vi "Tornado.vi"(11 "VI Ref":refnum<vi>) -> ()   [LabVIEW 2019]
doc: "Tornado disaster. A tornado appears on the left edge of the screen and then travels right across the screen. It will place any objects it passes close by into a spin, messing up block diagram wiring. There's also a 15% chance it will destroy an object on contact."
uses:
  _Sound/Music Player Command Message.ctl
  _Sound/Music Player Command.ctl
  _2D/Point.ctl
  <vilib>/Utility/miscctls.llb/LVRectTypeDef.ctl
  <vilib>/Utility/miscctls.llb/LVPositionTypeDef.ctl
  _SubVIs/Tornado State Enum.ctl
  <vilib>/numeric/Random Number (Range) U64.vi
  <vilib>/numeric/Random Number (Range) I64.vi
  <vilib>/numeric/Random Number (Range) DBL.vi
  <vilib>/numeric/sub_Random U32.vi
  _Window/Window.lvlib
  _Sound/Sound.lvlib
  _2D/2D.lvlib
panel:
  out "Tornado":u16(ring)
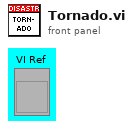
[diagram p1: front panel]
types:
  T1 = typedef "Tornado State Enum.ctl" = enum16{"Init", "Init Window", "Play Music", "Fade In Window", "Update Time", "Update Window Position", "Check Window Over BD", "Object Collision Detection", "Move Objects", "Update Graphic", "Fade Out Window", "Close Window"}
  T2 = typedef "LVPositionTypeDef.ctl" = cluster{"Left":i32, "Top":i32}
  T3 = cluster{"Object Ref":refnum<vi>, "hWnd":i32, "Initial Time (s)":dbl, "Release Time (s)":dbl, "Center Position":T2, "Start Position":T2, "Spin Velocity":dbl}[]
  T4 = enum32{"Invalid", "Standard", "Closed", "Hidden", "Minimized", "Maximized"}
  T5 = typedef "LVRectTypeDef.ctl" = cluster{"Left":i16, "Top":i16, "Right":i16, "Bottom":i16}
  T6 = typedef "2D.lvlib/Point.ctl" = cluster{"X":i16, "Y":i16}
  T7 = typedef "Sound.lvlib/Music Player Command Message.ctl" = cluster{"Command":T8, "Data":variant}
  T8 = typedef "Sound.lvlib/Music Player Command.ctl" = enum16{"Enable", "Play", "Play Random", "Stop", "Shutdown"}
  T9 = cluster{"Object Ref":refnum<vi>, "hWnd":i32, "Initial Time (s)":dbl, "Release Time (s)":dbl, "Center Position":T2, "Start Position":T2, "Spin Velocity":dbl}
  T10 = cluster{"BDWin.NativeWindow":u64, "vi reference":refnum<vi>}[]
  T11 = typedef "LVPointTypeDef.ctl" = cluster{"Horizontal":i16, "Vertical":i16}
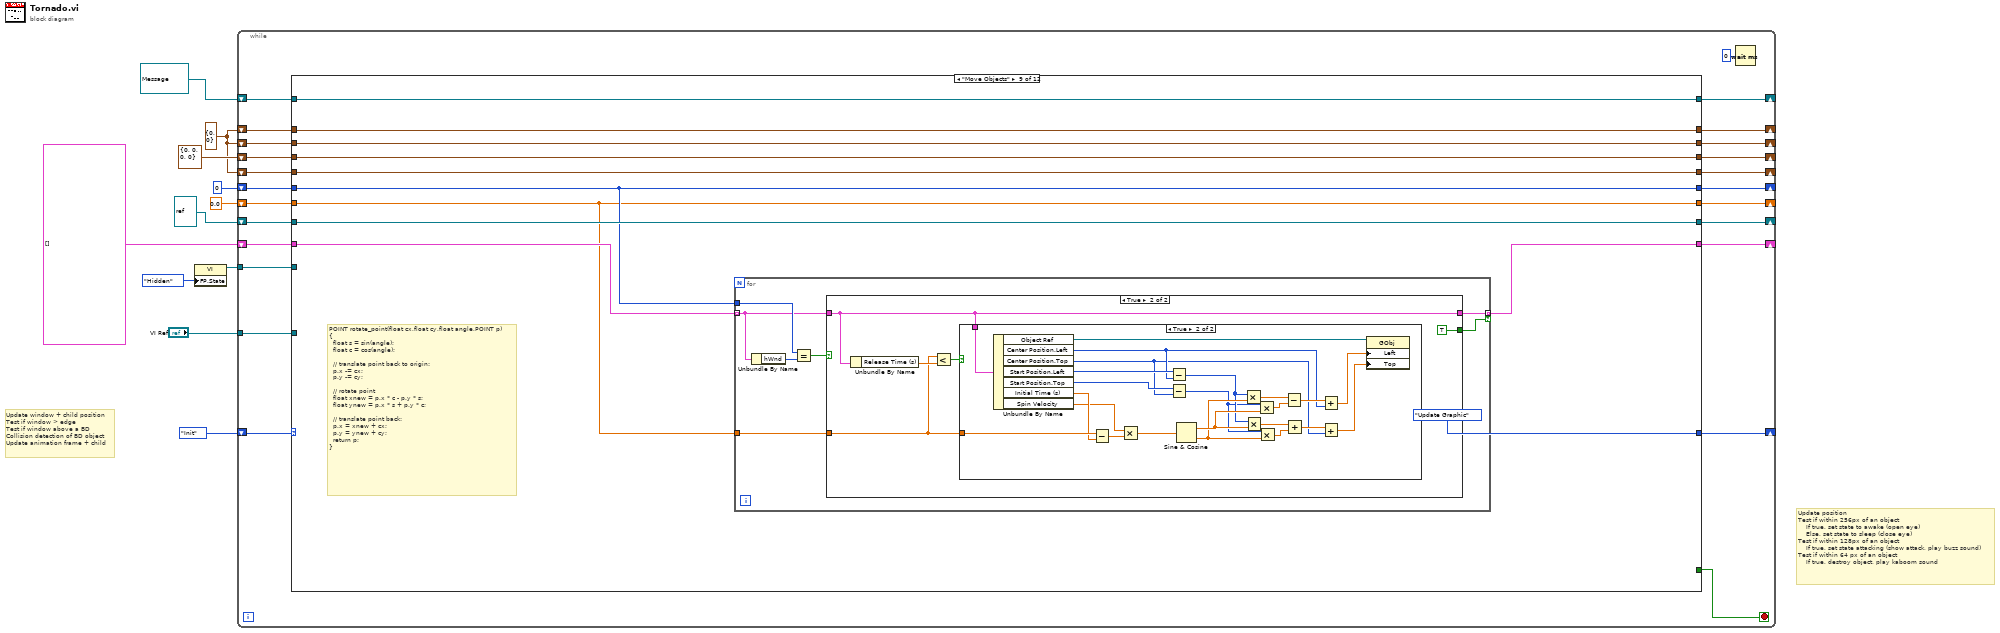
[diagram p0: block diagram]
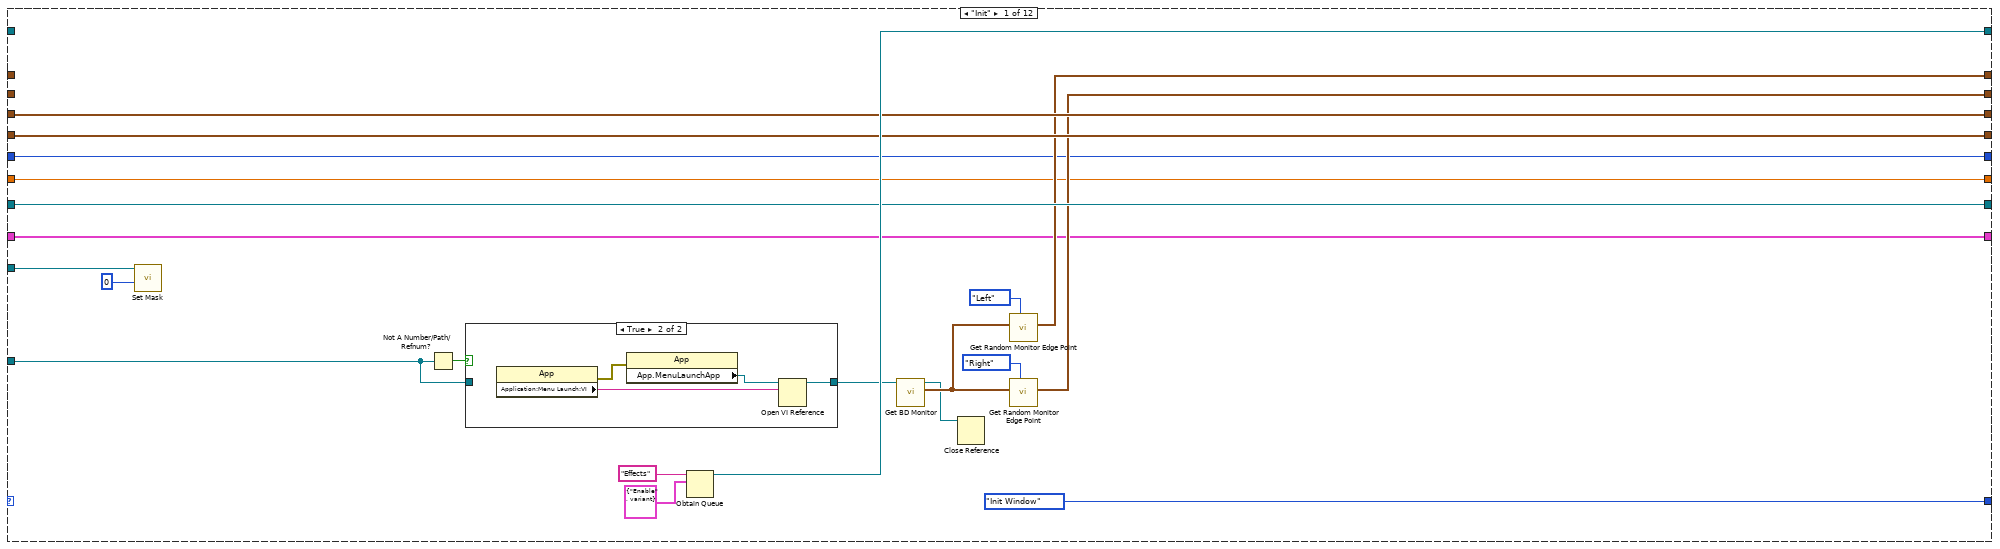
[diagram p2: hidden frame]
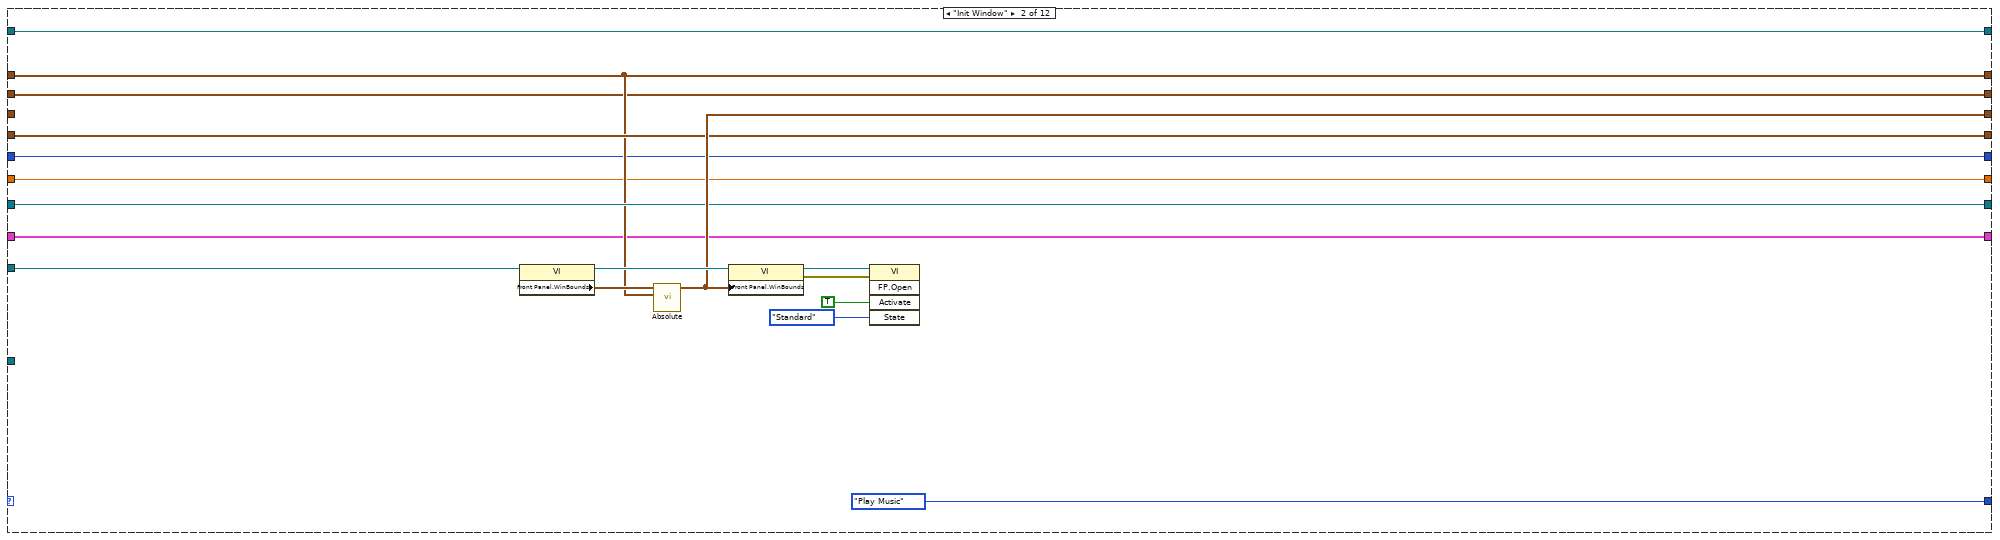
[diagram p4: hidden frame]
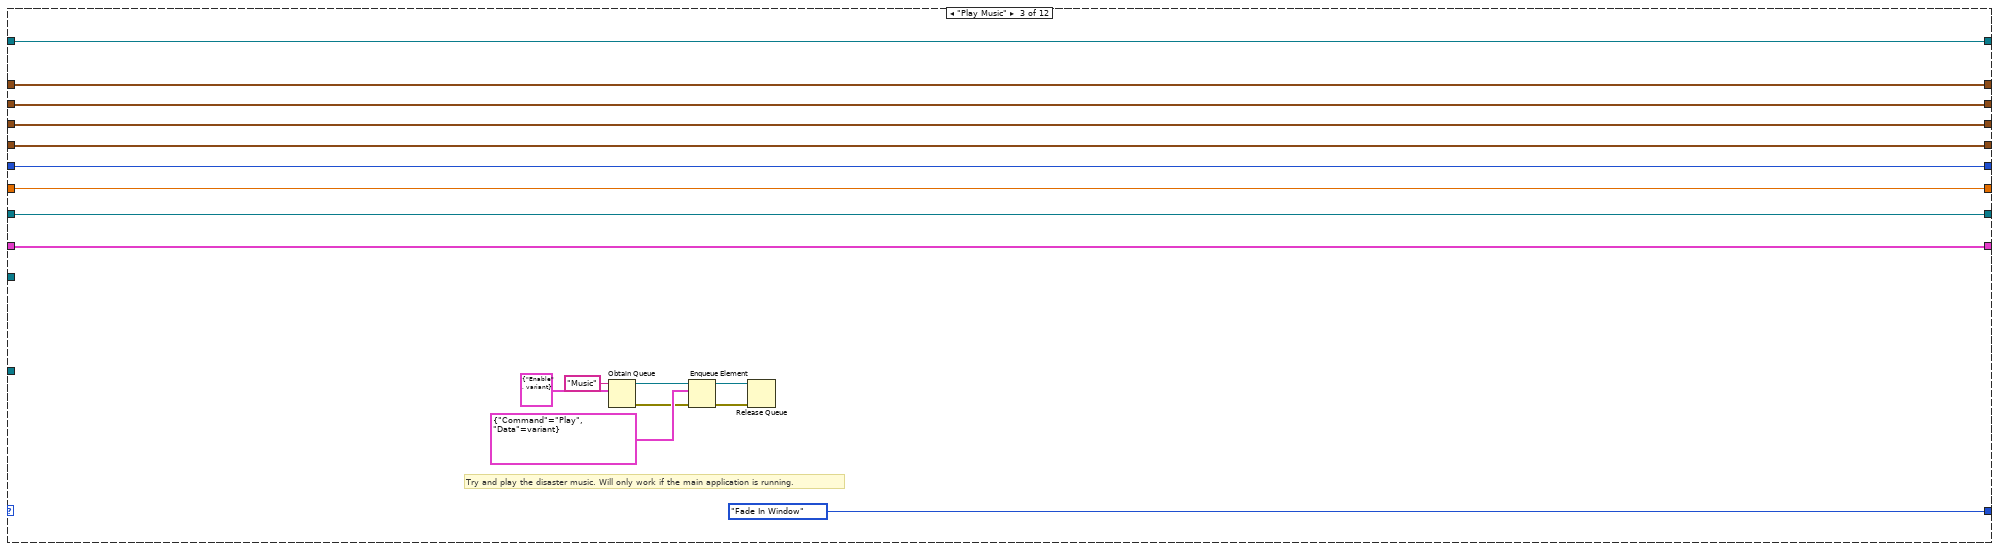
[diagram p5: hidden frame]
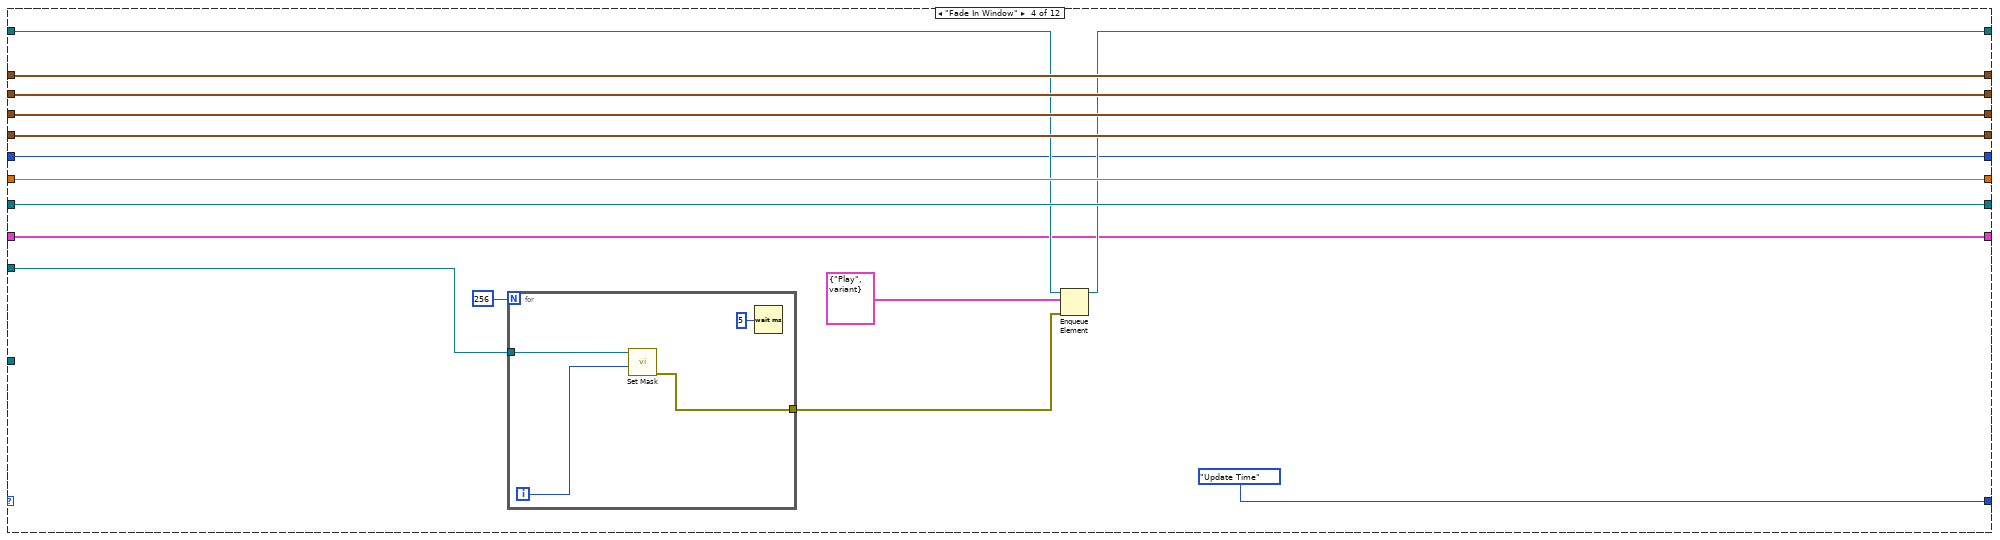
[diagram p6: hidden frame]
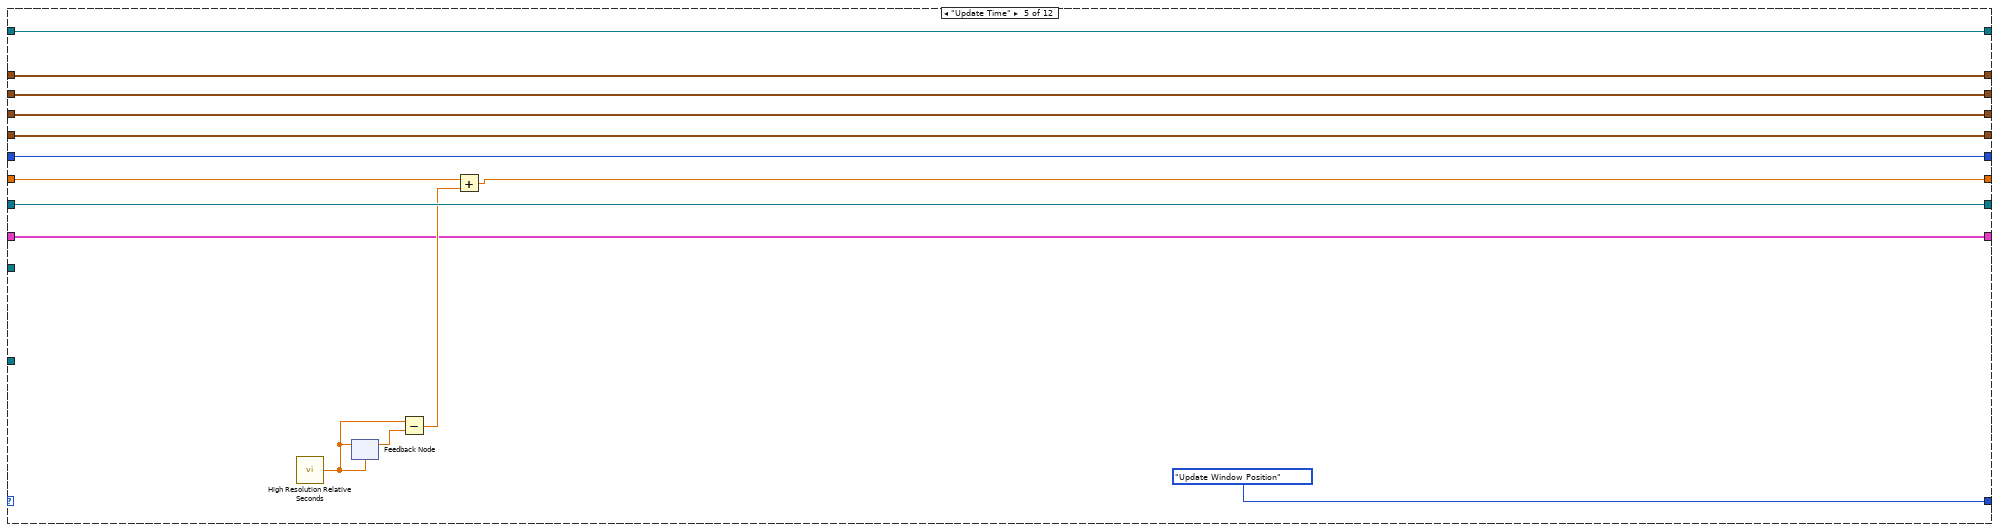
[diagram p7: hidden frame]
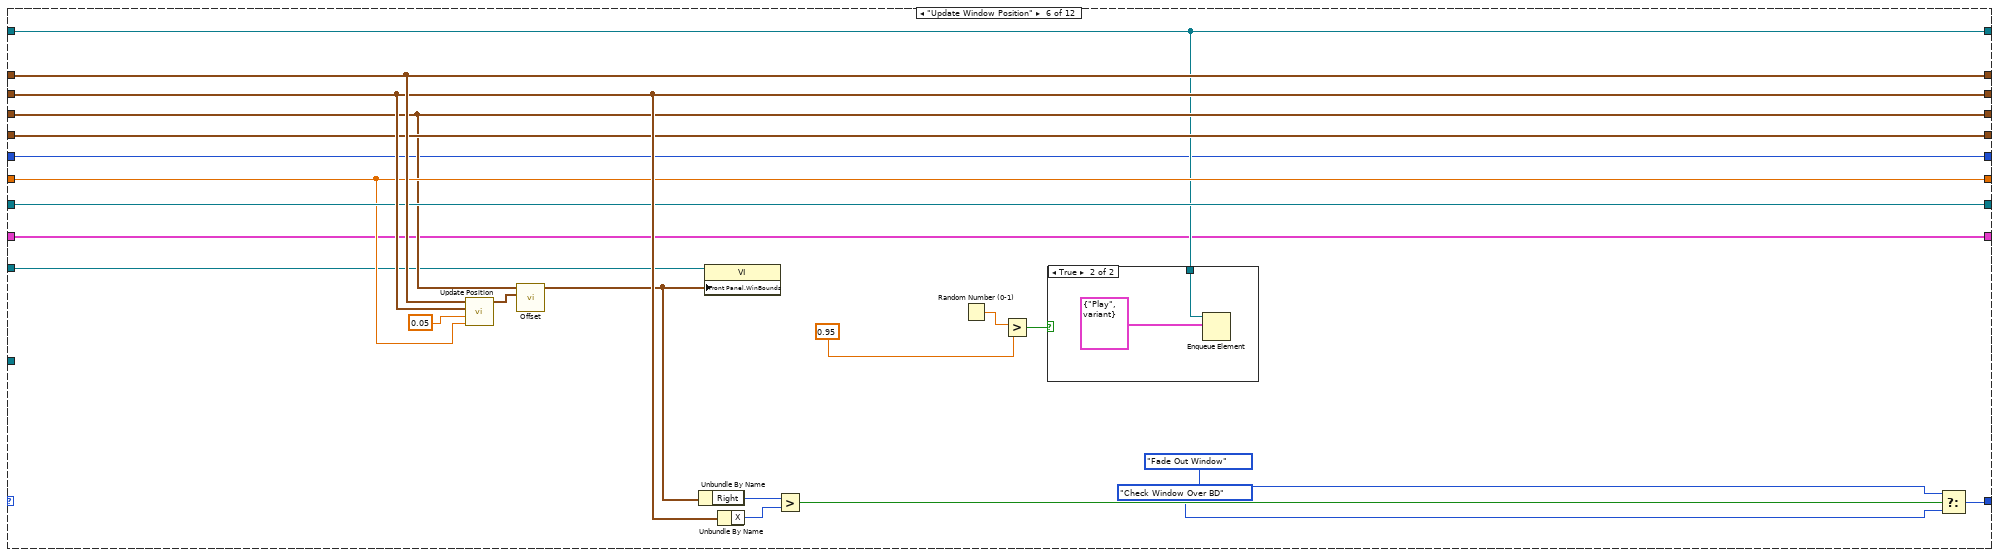
[diagram p8: hidden frame]
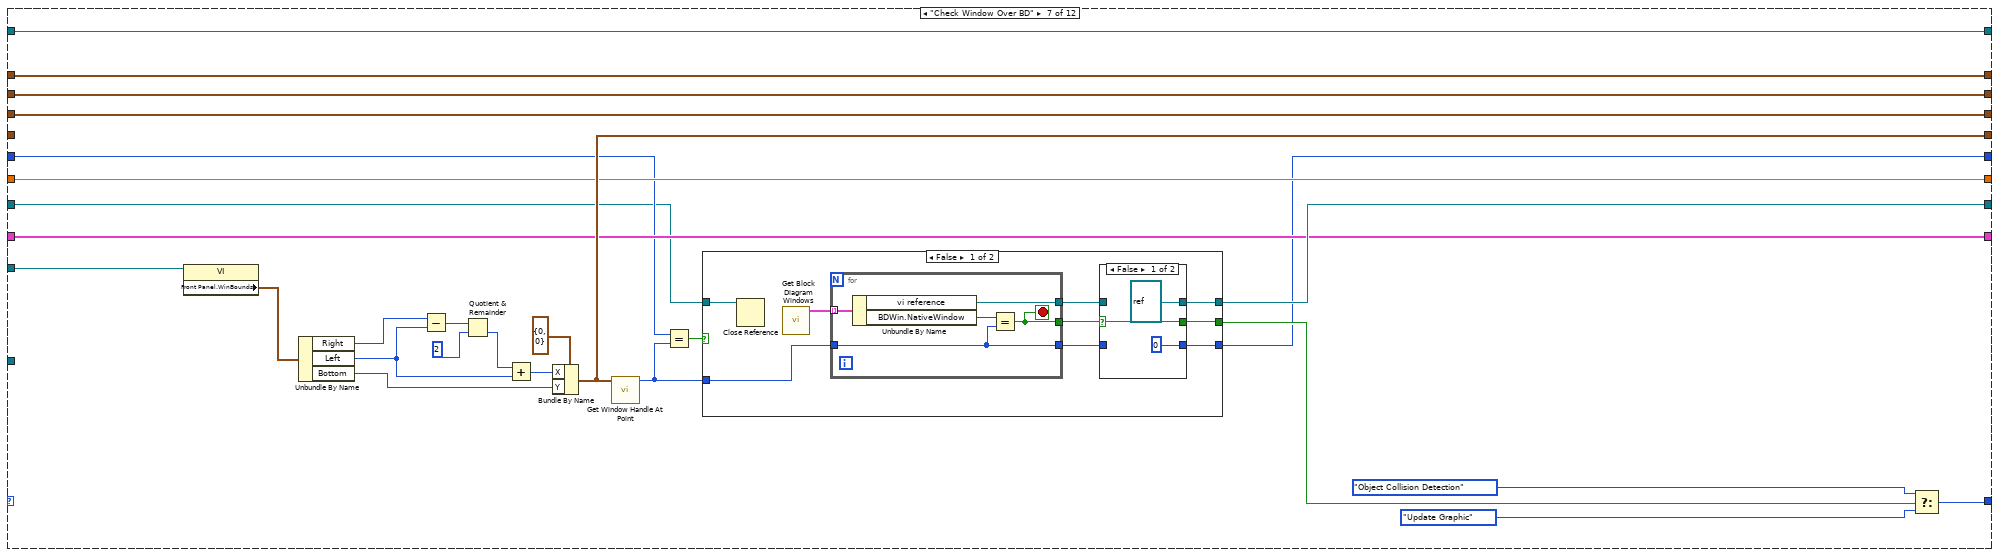
[diagram p10: hidden frame]
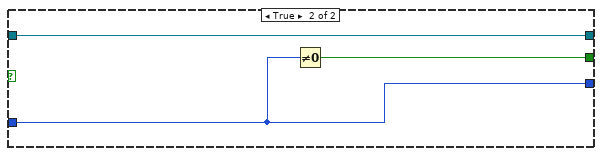
[diagram p12: hidden frame]
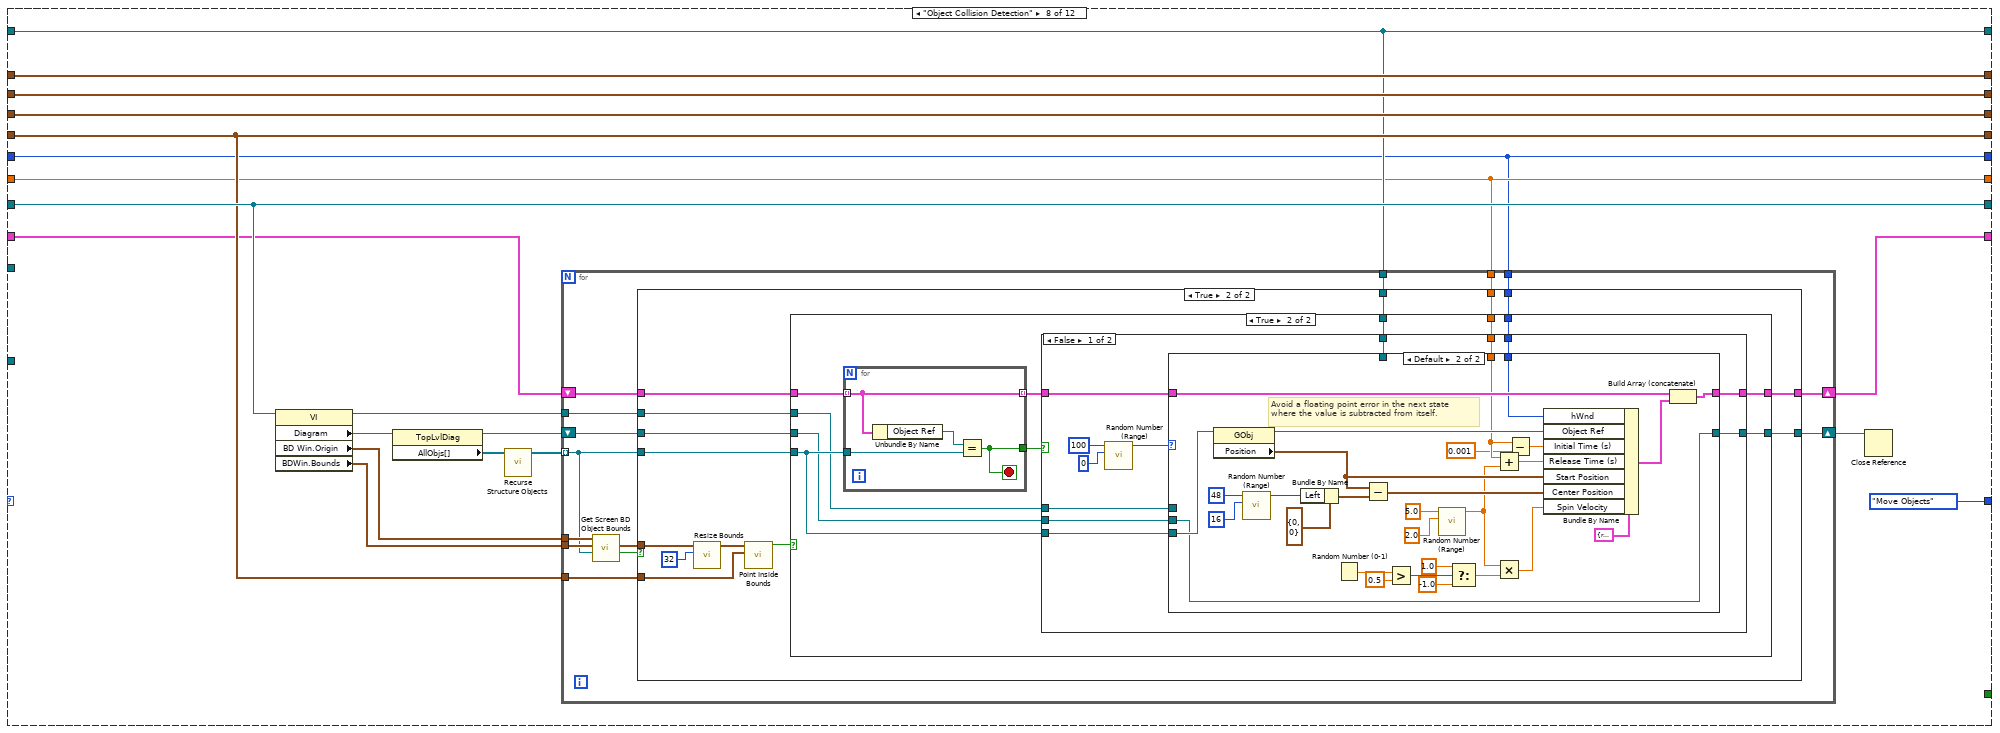
[diagram p13: hidden frame]
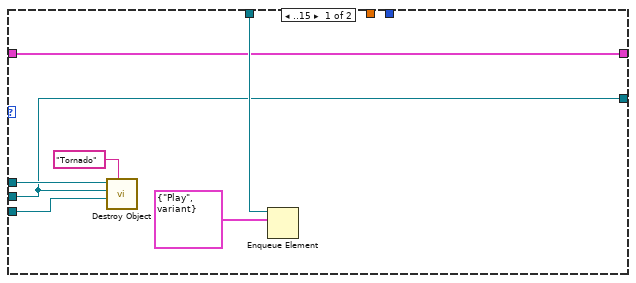
[diagram p16: hidden frame]
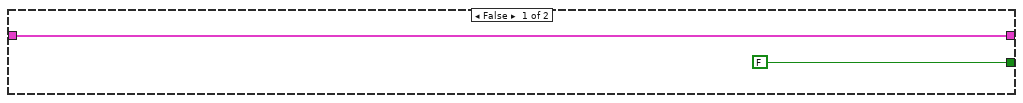
[diagram p18: hidden frame]
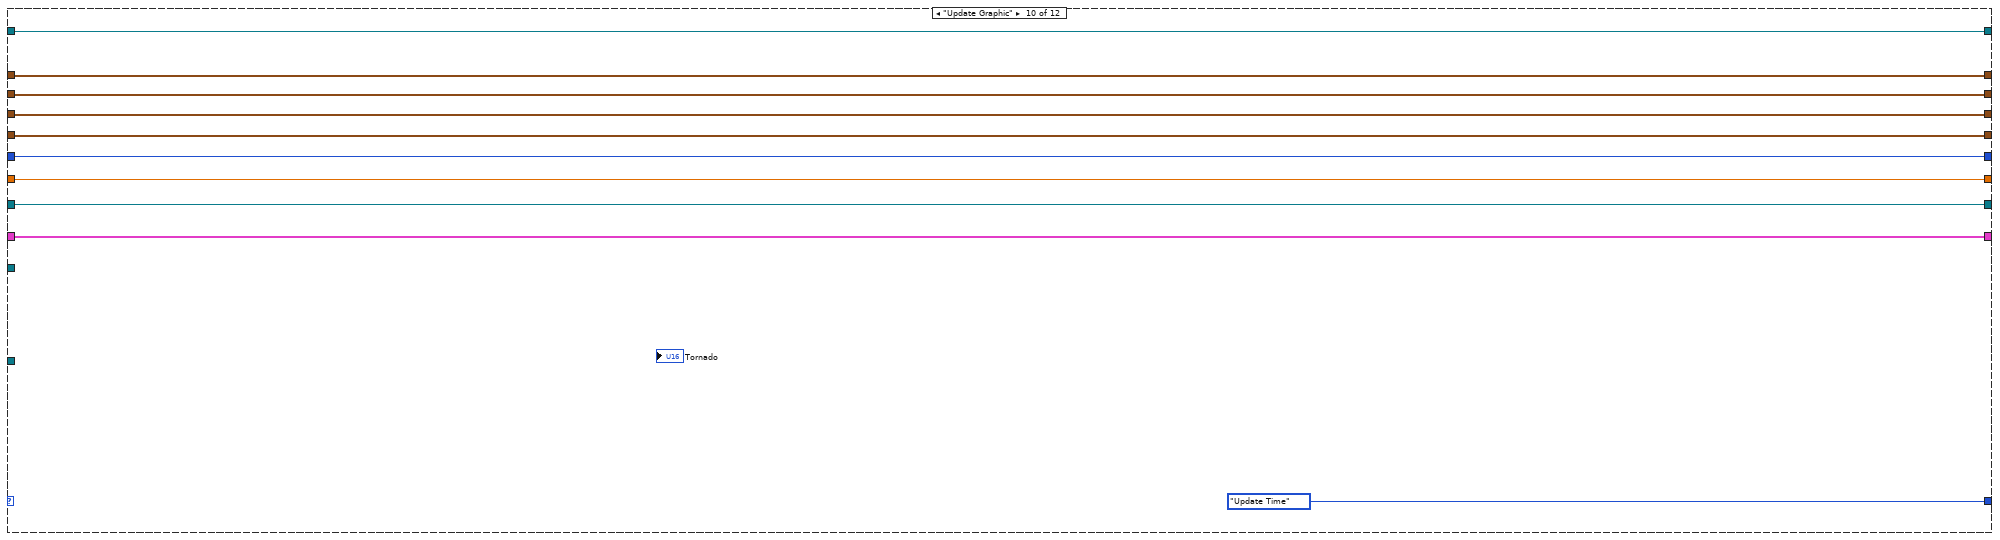
[diagram p20: hidden frame]
diagram:
  w8 = T6 {"X"=0, "Y"=0} ("Point")
  # "Update position\nTest if within 256px of an object\n    If true, set state to awake (open eye)\n    Else, set state to sleep (close eye)\nTest if within 128px of an object\n    If true, set state attacking (show attack, play buzz sound)\nTest if within 64 px of an object\n    If true, destroy object, play kaboom sound"
  # "Update window + child position\nTest if window > edge\nTest if window above a BD\nCollision detection of BD object\nUpdate animation frame + child"
  n1 = property class="VI"("FP.State"=T4."Hidden" ("Front Panel Window:State")) -> (reference out=w5:refnum<vi>)  [unwired: 2 in, 1 out]
  n2 = while {
    shift-right: [w32] -> _
    shift-left: Tornado_State_Enum."Init" ("Enum") -> [w35]
    tunnel: w5 -> [w31]
    shift-right: [w33] -> _
    shift-left: refnum<queue> refnum ("queue out") -> [w30]
    shift-right: [w29] -> _
    shift-left: w8 -> [w27]
    shift-right: [w28] -> _
    shift-left: w8 -> [w26]
    shift-right: [w25] -> _
    shift-left: T5 {"Left"=0, "Top"=0, "Right"=0, "Bottom"=0} ("Bounds Out") -> [w24]
    shift-right: [w23] -> _
    shift-left: refnum<vi> refnum ("vi reference") -> [w20]
    shift-right: [w22] -> _
    shift-left: w8 -> [w21]
    tunnel: "VI Ref" -> [w34]
    shift-right: [w17] -> _
    shift-left: 0.0 -> [w18]
    shift-right: [w14] -> _
    shift-left: T3 [] -> [w15]
    shift-right: [w13] -> _
    shift-left: 0 ("hWnd") -> [w12]
    stop <- w19 stop-if-true
    n3 = case shown="\"Move Objects\"" w35 {
      tunnel: w34 -> [w54 _ _ _ _ _ _ _ _ _ _ _]
      tunnel: [w52 w72 w89 w101 w128 w133 w179 w209 w329 w376 w388 refnum<queue> refnum ("queue out")] -> w33
      tunnel: [Tornado_State_Enum."Init Window" ("Enum") Tornado_State_Enum."Play Music" ("Enum") Tornado_State_Enum."Fade In Window" ("Enum") Tornado_State_Enum."Update Time" ("Enum") Tornado_State_Enum."Update Window Position" ("Enum") w144 w164 Tornado_State_Enum."Move Objects" ("Enum") Tornado_State_Enum."Update Graphic" ("Enum") Tornado_State_Enum."Update Time" ("Enum") Tornado_State_Enum."Close Window" ("Enum") Tornado_State_Enum."Close Window" ("Enum")] -> w32
      tunnel: w31 -> [w40 w73 _ w104 _ w138 w167 _ _ _ w381 w404]
      tunnel: w30 -> [_ w72 w89 w100 w128 w133 w179 w209 w329 w376 w388 w403]
      tunnel: [w44 w68 w88 w109 w127 w146 w178 w221 w328 w375 w387 w408] -> w29
      tunnel: [w43 w67 w87 w108 w126 w143 w177 w220 w327 w374 w386 w407] -> w28
      tunnel: w27 -> [_ w68 w88 w109 w127 w146 w178 w221 w328 w375 w387 w408]
      tunnel: w26 -> [_ w67 w87 w108 w126 w143 w177 w220 w327 w374 w386 w407]
      tunnel: [w51 w71 w86 w107 w125 w139 w176 w219 w326 w373 w385 w406] -> w25
      tunnel: w24 -> [w51 _ w86 w107 w125 w139 w176 w219 w326 w373 w385 w406]
      tunnel: [w49 w69 w84 w105 w124 w141 w163 w213 w325 w372 w384 refnum<vi> refnum ("vi reference")] -> w23
      tunnel: [w50 w70 w85 w106 w123 w142 w162 w212 w320 w371 w383 w405] -> w22
      tunnel: w21 -> [w50 w70 w85 w106 w123 w142 _ w212 w320 w371 w383 w405]
      tunnel: w20 -> [w49 w69 w84 w105 w124 w141 w153 w213 w325 w372 w384 w396]
      tunnel: [_ _ _ _ _ _ _ _ _ _ _ TRUE] -> w19
      tunnel: w18 -> [w42 w66 w83 w103 w121 w140 w161 w208 w319 w370 w380 w400]
      tunnel: [w42 w66 w83 w103 w118 w140 w161 w208 w319 w370 w380 w400] -> w17
      tunnel: w15 -> [w39 w64 w82 w98 w117 w132 w160 w206 w322 w369 w379 w399]
      tunnel: [w39 w64 w82 w98 w117 w132 w160 w207 w321 w369 w379 w399] -> w14
      tunnel: [w37 w62 w80 w96 w115 w129 w157 w204 w323 w367 w377 w397] -> w13
      tunnel: w12 -> [w37 w62 w80 w96 w115 w129 w156 w204 w323 w367 w377 w397]
      frame "Init" {
        n4 = call "Set Mask.vi"("Alpha (255)"=0, "VI Ref In"=w40) -> ()  [unwired: 8 in, 2 out]
        n5 = Not A Number/Path/Refnum?(number/path/refnum=w54) -> (NaN/Path/Refnum?=w53:bool)
        n6 = case shown="True" w53 {
          tunnel: w54 -> [w57 _]
          tunnel: [w57 w60] -> w45
          frame False {
          }
          frame True {
            n7 = property class="App"() -> (error out=w59:errorcluster, "Application:Menu Launch:VI"=w61:string)  [unwired: 2 in, 1 out]
            n8 = property class="App"(error in=w59) -> ("App.MenuLaunchApp"=w58:refnum<vi>)  [unwired: 1 in, 2 out]
            n9 = Open VI Reference(application reference (local)=w58, vi path=w61) -> (vi reference=w60:refnum<vi>)  [unwired: 4 in, 1 out]
          }
        }
        n10 = Obtain Queue(name (unnamed)="Effects", element data type=T7 {"Command"=enum."Enable", "Data"=variant} ("Message")) -> (queue out=w52:refnum<queue>)  [unwired: 3 in, 2 out]
        n11 = call "Get BD Monitor.vi"("VI Ref In"=w45) -> ("Monitor Bounds"=w48:T5, "VI Ref Out"=w36:refnum<vi>)  [unwired: 8 in, 1 out]
        n12 = Close Reference(reference=w36) -> ()  [unwired: 1 in, 1 out]
        n13 = call "Get Random Monitor Edge Point.vi"("Edge"=enum16{"Left", "Top", "Right", "Bottom"}."Left", "Monitor Bounds"=w48) -> ("Point"=w44:T6)  [unwired: 9 in]
        n14 = call "Get Random Monitor Edge Point.vi"("Edge"=enum16{"Left", "Top", "Right", "Bottom"}."Right", "Monitor Bounds"=w48) -> ("Point"=w43:T6)  [unwired: 9 in]
      }
      frame "Init Window" {
        n15 = property class="VI"(reference=w73) -> (reference out=w76:refnum<vi>, "Front Panel.WinBounds"=w78:T5)  [unwired: 1 in, 1 out]
        n16 = call "Absolute.vi"("Point"=w68, "Bounds In"=w78) -> ("Bounds Out"=w71:T5)  [unwired: 9 in]
        n17 = property class="VI"(reference=w76, "Front Panel.WinBounds"=w71) -> (reference out=w77:refnum<vi>, error out=w65:errorcluster)  [unwired: 1 in]
        n18 = invoke class="VI" method="FP.Open"(reference=w77, error in=w65, "Activate"=TRUE ("Activate?"), "State"=T4."Standard") -> ()  [unwired: 1 in, 5 out]
      }
      frame "Play Music" {
        # "Try and play the disaster music. Will only work if the main application is running."
        n19 = Obtain Queue(name (unnamed)="Music", element data type=T7 {"Command"=enum."Enable", "Data"=variant} ("Message")) -> (queue out=w92:refnum<queue>, error out=w79:errorcluster)  [unwired: 3 in, 1 out]
        n20 = Enqueue Element(queue=w92, element=T7 {"Command"=enum."Play", "Data"=variant(string "Disasters\\Disaster Decision")}, error in (no error)=w79) -> (queue out=w91:refnum<queue>, error out=w90:errorcluster)  [unwired: 1 in, 1 out]
        n21 = Release Queue(queue=w91, error in (no error)=w90) -> ()  [unwired: 1 in, 3 out]
      }
      frame "Fade In Window" {
        n22 = for {
          N: 256 -> [_]
          tunnel: w104 -> [w112]
          tunnel: [w111] -> w99
          i -> [w113]
          n23 = call "Set Mask.vi"("Alpha (255)"=w113, "VI Ref In"=w112) -> ("error out"=w111:errorcluster)  [unwired: 8 in, 1 out]
          n24 = Wait (ms)(milliseconds to wait=u32 5) -> ()  [unwired: 1 out]
        }
        n25 = Enqueue Element(queue=w100, element=T7 {"Command"=enum."Play", "Data"=variant(string "siren")}, error in (no error)=w99) -> (queue out=w101:refnum<queue>)  [unwired: 1 in, 2 out]
      }
      frame "Update Time" {
        n26 = call <vilib>:"High Resolution Relative Seconds.vi"() -> ("relative seconds"=w119:dbl)
        n27 = feedback-in #1(w119) -> ()
        n28 = feedback #1(w119) -> (w122:dbl)
        n29 = Subtract(x=w119, y=w122) -> (x-y=w120:dbl)
        n30 = Add(x=w121, y=w120) -> (x+y=w118:dbl)
      }
      frame "Update Window Position" {
        n31 = call "Update Position.vi"("Time"=w140, "Speed"=0.05 ("Speed (px/sec)"), "End Pos"=w143, "Start Pos"=w146) -> ("Current Pos"=w148:T6)  [unwired: 7 in]
        n32 = call "Offset.vi"("Point"=w148, "Bounds In"=w139) -> ("Bounds Out"=w137:T5)  [unwired: 9 in]
        n33 = Unbundle By Name(w137) -> ("Right"=w150:i16)
        n34 = property class="VI"(reference=w138, "Front Panel.WinBounds"=w137) -> ()  [unwired: 1 in, 2 out]
        n35 = Unbundle By Name(w143) -> ("X"=w149:i16)
        n36 = Greater?(x=w150, y=w149) -> (0:w145:bool)
        n37 = Random Number (0-1)() -> (number: 0 to 1=w136:dbl)
        n38 = Greater?(x=w136, y=0.95) -> (0:w134:bool)
        n39 = case shown="True" w134 {
          tunnel: w133 -> [_ w151]
          frame False {
          }
          frame True {
            n40 = Enqueue Element(queue=w151, element=T7 {"Command"=enum."Play", "Data"=variant(string "wind")}) -> ()  [unwired: 2 in, 3 out]
          }
        }
        n41 = Select(t=Tornado_State_Enum."Fade Out Window" ("Enum"), s=w145, f=Tornado_State_Enum."Check Window Over BD" ("Enum")) -> (s? t:f=w144:T1)
      }
      frame "Check Window Over BD" {
        n42 = property class="VI"(reference=w167) -> ("Front Panel.WinBounds"=w166:T5)  [unwired: 1 in, 2 out]
        n43 = Unbundle By Name(w166) -> ("Right"=w175:i16, "Left"=w171:i16, "Bottom"=w168:i16)
        n44 = Subtract(x=w175, y=w171) -> (x-y=w174:i16)
        n45 = Quotient & Remainder(x=w174, y=i16 2) -> (floor(x/y)=w172:i16)  [unwired: 1 out]
        n46 = Add(x=w172, y=w171) -> (x+y=w169:i16)
        n47 = Bundle By Name(cluster=T6 {"X"=0, "Y"=0} ("Point"), "X"=w169, "Y"=w168) -> (w162:T6)
        n48 = call "Get Window Handle At Point.vi"("Point"=w162) -> ("hWnd"=w155:i32)  [unwired: 9 in, 1 out]
        n49 = Equal?(x=w156, y=w155) -> (x = y?=w154:bool)
        n50 = case shown="False" w154 {
          tunnel: w155 -> [w187 w200]
          tunnel: [w184 w201] -> w165
          tunnel: [w181 w202] -> w163
          tunnel: [w180 w200] -> w157
          tunnel: w153 -> [w186 w202]
          frame False {
            n51 = Close Reference(reference=w186) -> ()  [unwired: 1 in, 1 out]
            n52 = call "Get Block Diagram Windows.vi"() -> ("VIs With Open BDs"=w188:T10)  [unwired: 11 in]
            n53 = for {
              tunnel: w188 -> [w199] mode=indexing
              tunnel: [w198] -> w182
              tunnel: [w197] -> w185
              tunnel: w187 -> [w195]
              tunnel: [w195] -> w183
              stop <- w197 stop-if-true
              n54 = Unbundle By Name(w199) -> ("vi reference"=w198:refnum<vi>, "BDWin.NativeWindow"=w196:u64)
              n55 = Equal?(x=w196, y=w195) -> (x = y?=w197:bool)
            }
            n56 = case shown="False" w185 {
              selector: w185 -> [w191 w194]
              tunnel: [w191 w194] -> w184
              tunnel: w183 -> [_ w192]
              tunnel: w182 -> [_ w193]
              tunnel: [refnum<vi> refnum ("vi reference") w193] -> w181
              tunnel: [0 ("hWnd") w192] -> w180
              frame False {
              }
              frame True {
              }
            }
          }
          frame True {
            n57 = Not Equal To 0?(x=w200) -> (x != 0?=w201:bool)
          }
        }
        n58 = Select(t=Tornado_State_Enum."Object Collision Detection" ("Enum"), s=w165, f=Tornado_State_Enum."Update Graphic" ("Enum")) -> (s? t:f=w164:T1)
      }
      frame "Object Collision Detection" {
        n59 = property class="VI"(reference=w213) -> (reference out=w215:refnum<vi>, "Diagram"=w217:refnum<vi>, "BD Win.Origin"=w211:T11, "BDWin.Bounds"=w210:T5)  [unwired: 1 in, 1 out]
        n60 = property class="TopLvlDiag"(reference=w217) -> (reference out=w214:refnum<vi>, "AllObjs[]"=w218:refnum<vi>[])  [unwired: 1 in, 1 out]
        n61 = call "Recurse Structure Objects.vi"("Objects In"=w218) -> ("Objects Out"=w216:refnum<vi>[])  [unwired: 10 in]
        n62 = for {
          tunnel: w211 -> [w235]
          tunnel: w210 -> [w234]
          tunnel: w216 -> [w229] mode=indexing
          tunnel: w212 -> [w231]
          tunnel: w215 -> [w230]
          tunnel: w209 -> [w227]
          shift-right: [w225] -> w207
          shift-left: w206 -> [w226]
          tunnel: w208 -> [w224]
          tunnel: w204 -> [w223]
          shift-right: [w222] -> w203
          shift-left: w214 -> [w228]
          n63 = call "Get Screen BD Object Bounds.vi"("Object Reference"=w229, "BD Window Bounds"=w234, "BD Origin"=w235) -> ("Object Visible?"=w233:bool, "Screen Object Bounds"=w232:T5)  [unwired: 6 in, 1 out]
          n64 = case shown="True" w233 {
            tunnel: w232 -> [_ w239]
            tunnel: w231 -> [_ w242]
            tunnel: w230 -> [_ w246]
            tunnel: w229 -> [_ w248]
            tunnel: w228 -> [w236 w247]
            tunnel: w227 -> [_ w245]
            tunnel: w226 -> [w237 w244]
            tunnel: [w237 w243] -> w225
            tunnel: w224 -> [_ w241]
            tunnel: w223 -> [_ w240]
            tunnel: [w236 w238] -> w222
            frame False {
            }
            frame True {
              n65 = call "Resize Bounds.vi"("Resize Amount"=i16 32, "Bounds In"=w239) -> ("Bounds Out"=w250:T5)  [unwired: 9 in]
              n66 = call "Point Inside Bounds.vi"("Point"=w242, "Bounds"=w250) -> ("Inside?"=w249:bool)  [unwired: 9 in]
              n67 = case shown="True" w249 {
                tunnel: w248 -> [_ w260]
                tunnel: w247 -> [w252 w256]
                tunnel: w246 -> [_ w257]
                tunnel: w245 -> [_ w255]
                tunnel: w244 -> [w253 w264]
                tunnel: [w253 w263] -> w243
                tunnel: w241 -> [_ w262]
                tunnel: w240 -> [_ w261]
                tunnel: [w252 w254] -> w238
                frame False {
                }
                frame True {
                  n68 = for {
                    tunnel: w264 -> [w317] mode=indexing
                    tunnel: w260 -> [w318]
                    tunnel: [w317] -> w258 mode=indexing
                    tunnel: [w316] -> w259
                    stop <- w316 stop-if-true
                    n69 = Unbundle By Name(w317) -> ("Object Ref"=w315:refnum<vi>)
                    n70 = Equal?(x=w315, y=w318) -> (x = y?=w316:bool)
                  }
                  n71 = case shown="False" w259 {
                    tunnel: w258 -> [w276 w314]
                    tunnel: w260 -> [w272 _]
                    tunnel: [w275 w314] -> w263
                    tunnel: w262 -> [w273 _]
                    tunnel: w261 -> [w274 _]
                    tunnel: w257 -> [w271 _]
                    tunnel: w256 -> [w270 w313]
                    tunnel: w255 -> [w269 _]
                    tunnel: [w265 w313] -> w254
                    frame False {
                      n72 = call-poly <vilib>:"Random Number (Range).vi"("lower bound (0)"=u64 0, "upper bound (100)"=u64 100) -> ("number"=w266:u64)  [unwired: 9 in]
                      n73 = case shown="Default" w266 {
                        tunnel: w276 -> [w278 w312]
                        tunnel: [w278 w311] -> w275
                        tunnel: w274 -> [_ w307]
                        tunnel: w273 -> [_ w295]
                        tunnel: w272 -> [w280 w304]
                        tunnel: w271 -> [w281 _]
                        tunnel: w270 -> [w277 w284]
                        tunnel: w269 -> [w279 _]
                        tunnel: [w277 w284] -> w265
                        frame ..15 {
                          n74 = call "Destroy Object.vi"("Undo Text"="Tornado", "Object Ref"=w280, "BD Ref"=w277, "VI Ref"=w281) -> ()  [unwired: 7 in, 1 out]
                          n75 = Enqueue Element(queue=w279, element=T7 {"Command"=enum."Play", "Data"=variant(string "kaboom")}) -> ()  [unwired: 2 in, 3 out]
                        }
                        frame Default {
                          # "Avoid a floating point error in the next state where the value is subtracted from itself."
                          n76 = property class="GObj"(reference=w304) -> (reference out=w305:refnum<vi>, "Position"=w302:T2)  [unwired: 1 in, 1 out]
                          n77 = call-poly <vilib>:"Random Number (Range).vi"("lower bound (-100)"=i64 16 ("lower bound (0)"), "upper bound (100)"=i64 48) -> ("number"=w298:i64)  [unwired: 9 in]
                          n78 = Bundle By Name(cluster=T2 {"Left"=0, "Top"=0} ("y"), "Left"=w298) -> (w297:T2)
                          n79 = Random Number (0-1)() -> (number: 0 to 1=w292:dbl)
                          n80 = Subtract(x=w302, y=w297) -> (x-y=w303:T2)
                          n81 = Greater?(x=w292, y=0.5) -> (0:w290:bool)
                          n82 = call-poly <vilib>:"Random Number (Range).vi"("lower bound (0)"=2.0, "upper bound (100)"=5.0) -> ("number"=w288:dbl)  [unwired: 9 in]
                          n83 = Select(t=1.0, s=w290, f=-1.0) -> (s? t:f=w289:dbl)
                          n84 = Add(x=w295, y=w288) -> (x+y=w306:dbl)
                          n85 = Multiply(x=w288, y=w289) -> (x*y=w287:dbl)
                          n86 = Subtract(x=w295, y=0.001) -> (x-y=w293:dbl)
                          n87 = Bundle By Name(cluster=T9 {"Object Ref"=refnum, "hWnd"=0, "Initial Time (s)"=0.0, "Release Time (s)"=0.0, "Center Position"={"Left"=0, "Top"=0}, "Start Position"={"Left"=0, "Top"=0}, "Spin Velocity"=0.0}, "hWnd"=w307, "Object Ref"=w305, "Initial Time (s)"=w293, "Release Time (s)"=w306, "Start Position"=w302, "Center Position"=w303, "Spin Velocity"=w287) -> (w308:T9)
                          n88 = Build Array (concatenate)(w312, w308) -> (w311:T3)
                        }
                      }
                    }
                    frame True {
                    }
                  }
                }
              }
            }
          }
        }
        n89 = Close Reference(reference=w203) -> ()  [unwired: 1 in, 1 out]
      }
      frame "Move Objects" {
        # "POINT rotate_point(float cx,float cy,float angle,POINT p)\n{\n  float s = sin(angle);\n  float c = cos(angle);\n\n  // translate point back to origin:\n  p.x -= cx;\n  p.y -= cy;\n\n  // rotate point\n  float xnew = p.x * c - p.y * s;\n  float ynew = p.x * s + p.y * c;\n\n  // translate point back:\n  p.x = xnew + cx;\n  p.y = ynew + cy;\n  return p;\n}"
        n90 = for {
          tunnel: w322 -> [w333] mode=indexing
          tunnel: w323 -> [w336]
          tunnel: [w332] -> w321 mode=indexing if=w331
          tunnel: w319 -> [w330]
          n91 = Unbundle By Name(w333) -> ("hWnd"=w335:i32)
          n92 = Equal?(x=w336, y=w335) -> (x = y?=w334:bool)
          n93 = case shown="True" w334 {
            tunnel: w333 -> [w337 w340]
            tunnel: [w337 w340] -> w332
            tunnel: [FALSE TRUE] -> w331
            tunnel: w330 -> [_ w339]
            frame False {
            }
            frame True {
              n94 = Unbundle By Name(w340) -> ("Release Time (s)"=w342:dbl)
              n95 = Less?(x=w339, y=w342) -> (x < y?=w341:bool)
              n96 = case shown="True" w341 {
                tunnel: w340 -> [_ w366]
                tunnel: w339 -> [_ w365]
                frame False {
                }
                frame True {
                  n97 = Unbundle By Name(w366) -> ("Object Ref"=w352:refnum<vi>, "Center Position.Left"=w346:i32, "Center Position.Top"=w345:i32, "Start Position.Left"=w351:i32, "Start Position.Top"=w349:i32, "Initial Time (s)"=w364:dbl, "Spin Velocity"=w344:dbl)
                  n98 = Subtract(x=w365, y=w364) -> (x-y=w363:dbl)
                  n99 = Multiply(x=w344, y=w363) -> (x*y=w347:dbl)
                  n100 = Subtract(x=w351, y=w346) -> (x-y=w350:i32)
                  n101 = Subtract(x=w349, y=w345) -> (x-y=w348:i32)
                  n102 = Sine & Cosine(0:w347) -> (1:w358:dbl, 2:w357:dbl)
                  n103 = Multiply(x=w350, y=w357) -> (x*y=w362:dbl)
                  n104 = Multiply(x=w350, y=w358) -> (x*y=w359:dbl)
                  n105 = Multiply(x=w348, y=w358) -> (x*y=w361:dbl)
                  n106 = Multiply(x=w348, y=w357) -> (x*y=w360:dbl)
                  n107 = Subtract(x=w362, y=w361) -> (x-y=w356:dbl)
                  n108 = Add(x=w359, y=w360) -> (x+y=w354:dbl)
                  n109 = Add(x=w356, y=w346) -> (x+y=w355:dbl)
                  n110 = Add(x=w354, y=w345) -> (x+y=w353:dbl)
                  n111 = property class="GObj"(reference=w352, "Left"=w355, "Top"=w353) -> ()  [unwired: 1 in, 2 out]
                }
              }
            }
          }
        }
      }
      frame "Update Graphic" {
      }
      frame "Fade Out Window" {
        n112 = for {
          N: 256 -> [w393]
          tunnel: w381 -> [w389]
          i -> [w391]
          n113 = Decrement(x=w393) -> (x-1=w392:i32)
          n114 = Subtract(x=w392, y=w391) -> (x-y=w390:i32)
          n115 = call "Set Mask.vi"("Alpha (255)"=w390, "VI Ref In"=w389) -> ()  [unwired: 8 in, 2 out]
          n116 = Wait (ms)(milliseconds to wait=u32 5) -> ()  [unwired: 1 out]
        }
      }
      frame "Close Window" {
        n117 = invoke class="VI" method="FP.Close"(reference=w404) -> ()  [unwired: 2 in, 3 out]
        n118 = Close Reference(reference=w396) -> ()  [unwired: 1 in, 1 out]
        n119 = Release Queue(queue=w403) -> ()  [unwired: 2 in, 3 out]
      }
    }
    n120 = Wait (ms)(milliseconds to wait=u32 0) -> ()  [unwired: 1 out]
  }
